vi "Notify Event Complete.vi"(8 "error in (no error)":errorcluster, 10 "Completion Id":i64, 11 "Session in":refnum<class "Plugin Session.lvclass">) -> (0 "error out":errorcluster, 3 "Session out":refnum<class "Plugin Session.lvclass">)   [LabVIEW 2021, in "InstrumentStudio Plugin SDK.lvlib" / "Plugin Session.lvclass"]
doc: "Call this VI to notify the framework that the Project Saved event is complete. It is critical that the 'Notify Project Saved Event Complete.vi' is called in the Project Saved event so the framework does not hang"
uses:
  Plugin Session.lvclass
  Plugin Session.lvclass/Plugin Session.ctl
  Read Session Id.vi
  NationalInstruments.VIHost.Interop.dll
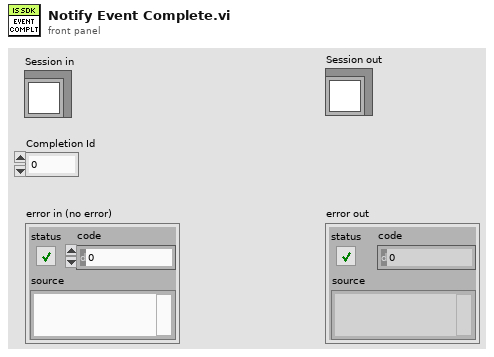
[diagram p1: front panel]
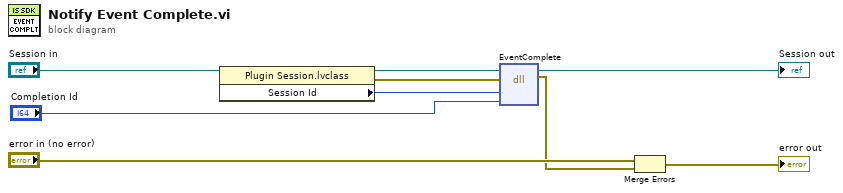
[diagram p0: block diagram]
diagram:
  n1 = property class="Plugin Session.lvclass"(reference="Session in") -> (reference out=→"Session out":refnum<class "Plugin Session.lvclass">, error out=w5:errorcluster, "Session Id"=w4:u64)  [unwired: 1 in]
  n2 = dll-call lib="C:/git/srd-adg-rf/dst/dstd/DSTInstStudio/source/utilities/PluginSDK/NationalInstruments.VIHost.Interop.dll" fn="EventComplete"(error in=w5, "hostId"=w4, "completionId"="Completion Id") -> (error out=w2:errorcluster)  [unwired: 5 in, 1 out]
  n3 = Merge Errors("error in (no error)", w2) -> (→"error out":errorcluster)
